vi "DAQ_PW_Read_Vdut_Vsource.vi"(8 "error in (no error)":errorcluster, 10 "DEV_BUSY":T1, 11 "DAQmx Device Name":tag) -> (1 "DAQmx Device Name ou":tag, 2 "Vsource":dbl format="%0.5f", 3 "JSON string":string)   [LabVIEW 2015]
uses:
  Share Data/uPower_kit.ctl
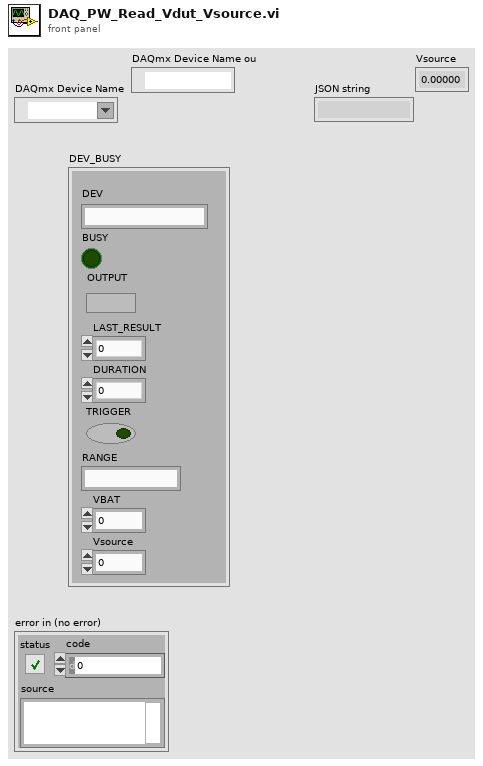
[diagram p1: front panel]
types:
  T1 = typedef "uPower_kit.ctl" = cluster{"DEV":string, "BUSY":bool, "VBAT":dbl, "OUTPUT":bool, "LAST_RESULT":dbl, "DURATION":u16, "TRIGGER":bool, "RANGE":string, "Vsource":dbl}
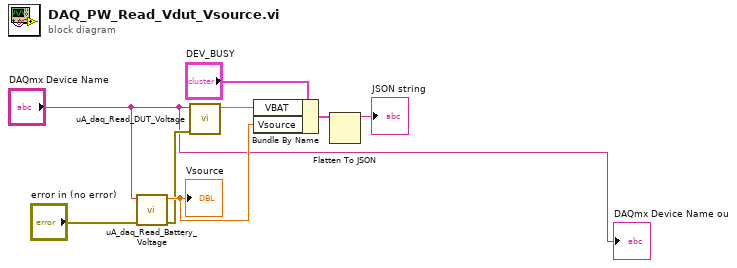
[diagram p0: block diagram]
diagram:
  n1 = call "uA_daq_Read_Battery_Voltage.vi"("error in"="error in (no error)", "USB DAQ"="DAQmx Device Name") -> ("error out"=w3:errorcluster, "Battery_Voltage"=w6:dbl)  [unwired: 8 in]
  "Vsource" <- w6
  n2 = call "uA_daq_Read_DUT_Voltage.vi"("error in"=w3, "USB DAQ"="DAQmx Device Name") -> ("DUT_Voltage"=w5:dbl)  [unwired: 8 in, 1 out]
  n3 = Bundle By Name(cluster="DEV_BUSY", "VBAT"=w5, "Vsource"=w6) -> (w7:T1)
  n4 = Flatten To JSON(anything=w7) -> (JSON string=→"JSON string":string)  [unwired: 2 in, 1 out]
  "DAQmx Device Name ou" <- "DAQmx Device Name"
